vi "ke_fit_gen_start.vi"(0 "Fitting parameters":T1={"A"=1.6, "B"=0.001, "C"=2200.0, "D"=-0.2} {"D" scale=-1.0..1.0; "C" scale=0.0..3000.0; "B" scale=0.0..0.002; "A" scale=0.0..2.0}, 7 "x array":i32[](array[numeric])) -> (4 "Fitting paramters array":dbl[](array[numeric]), 8 "y fit array":dbl[](array[numeric]))   [LabVIEW 2016]
doc: "This subvi generates a y fit array to the K E data from the LJ simulation. The input is the x array, which is just a sequential index list: 0,1,...Npts-1.\n\nThe fit is of the form: y=Aexp(-Bx)[sin(2*pi*x/C+D)]^2\n\nIt also outputs the four parameters as a simple 1D array with four values.\n\nPaul K Dixon\nP350\nCSUSB Physics"
uses:
  typedefs/fitting_parameters_for_ke.ctl
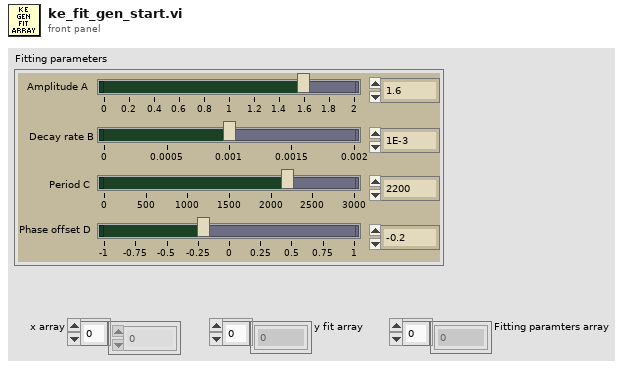
[diagram p1: front panel]
types:
  T1 = typedef "fitting_parameters_for_ke.ctl" = cluster{"A":dbl, "B":dbl, "C":dbl, "D":dbl}
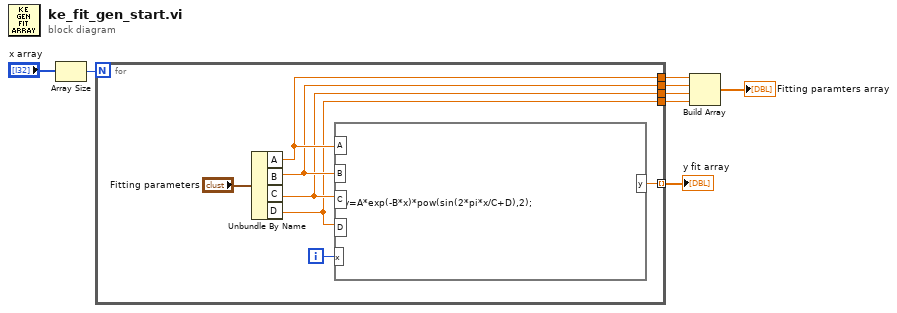
[diagram p0: block diagram]
diagram:
  n1 = Array Size(array="x array") -> (size(s)=w8:i32)
  n2 = for {
    N: w8 -> [_]
    tunnel: [w14] -> w6 mode=indexing
    tunnel: [w13] -> w5
    tunnel: [w12] -> w4
    tunnel: [w11] -> w3
    tunnel: [w10] -> w2
    i -> [w9]
    n3 = Unbundle By Name("Fitting parameters") -> ("A"=w13:dbl, "B"=w12:dbl, "C"=w11:dbl, "D"=w10:dbl)
    n4 = formula code="y=A*exp(-B*x)*pow(sin(2*pi*x/C+D),2);"("A"=w13, "B"=w12, "C"=w11, "D"=w10, "x"=w9) -> ("y"=w14:dbl)
  }
  "y fit array" <- w6
  n5 = Build Array(w5, w4, w3, w2) -> (→"Fitting paramters array":dbl[])
